vi "Pause.vi"(8 "Error In":errorcluster, 11 "Time(sec)":dbl) -> (0 "Error Out":errorcluster)   [LabVIEW 2017]
panel:
  # "PAUSE"
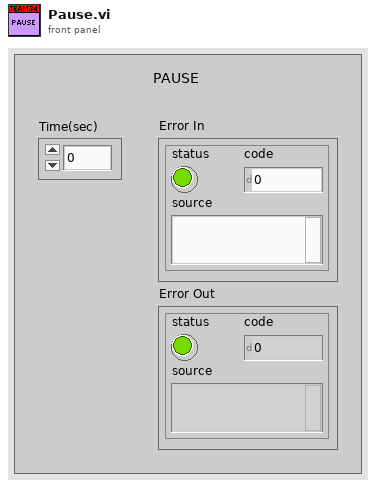
[diagram p1: front panel]
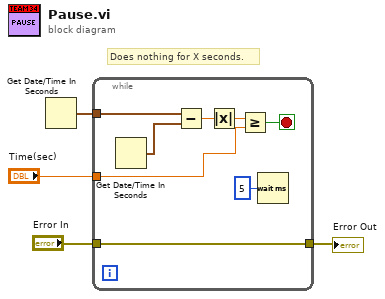
[diagram p0: block diagram]
diagram:
  # "Does nothing for X seconds."
  n1 = Get Date/Time In Seconds() -> (seconds since 1Jan1904=w4:timestamp)
  n2 = while {
    tunnel: w4 -> [w12]
    tunnel: "Time(sec)" -> [w6]
    tunnel: "Error In" -> [w5]
    tunnel: [w5] -> w1
    stop <- w8 stop-if-true
    n3 = Get Date/Time In Seconds() -> (seconds since 1Jan1904=w11:timestamp)
    n4 = Subtract(x=w12, y=w11) -> (x-y=w10:dbl)
    n5 = Absolute Value(x=w10) -> (abs(x)=w9:dbl)
    n6 = Greater Or Equal?(x=w9, y=w6) -> (x >= y?=w8:bool)
    n7 = Wait (ms)(milliseconds to wait=u32 5) -> ()  [unwired: 1 out]
  }
  "Error Out" <- w1
